vi "Test 3 Compatible Game.vi"(8 "error in (no error)":errorcluster, 11 "Test Case In":refnum<class "Game Test.lvclass">) -> (0 "error out":errorcluster, 3 "Test Case Out":refnum<class "Game Test.lvclass">)   [LabVIEW 2020, in "Game Test.lvclass"]
uses:
  Game Test.lvclass
  C:/Program Files (x86)/National Instruments/LabVIEW 2020/vi.lib/Astemes/LUnit/Test Case.lvclass
  Bag/Cubes.ctl
  <vilib>/Astemes/LUnit/Test Case.lvclass/Test Case.ctl
  <vilib>/Astemes/LUnit/Append Fail Result.vi
  <vilib>/Astemes/LUnit/Append Pass Result.vi
  Bag/Bag.lvclass
  <vilib>/Astemes/LUnit/Test Case.lvclass
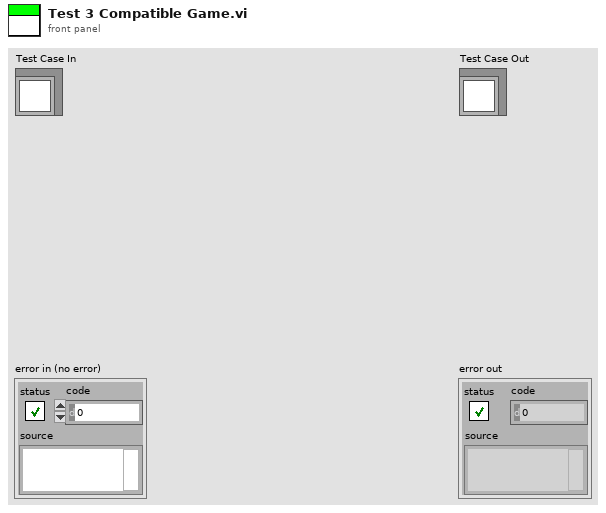
[diagram p1: front panel]
types:
  T1 = typedef "Bag.lvclass/Cubes.ctl" = cluster{"Red":i32, "Green":i32, "Blue":i32}
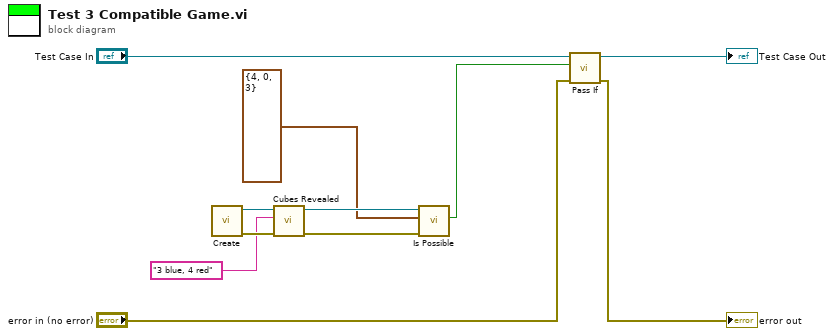
[diagram p0: block diagram]
diagram:
  n1 = call "Create.vi"() -> ("error out"=w6:errorcluster, "Bag"=w7:refnum<class "Bag.lvclass">)  [unwired: 10 in]
  n2 = call "Cubes Revealed.vi"("error in (no error)"=w6, "Set"="3 blue, 4 red", "Bag in"=w7) -> ("error out"=w3:errorcluster, "Bag out"=w4:refnum<class "Bag.lvclass">)  [unwired: 7 in]
  n3 = call "Is Possible.vi"("error in (no error)"=w3, "Cubes"=T1 {"Red"=4, "Green"=0, "Blue"=3}, "Bag in"=w4) -> ("Compatible?"=w1:bool)  [unwired: 6 in, 2 out]
  n4 = call <vilib>:"Pass If.vi"("error in (no error)"="error in (no error)", "Pass?"=w1, "LUnit Test Case In"="Test Case In") -> ("error out"=→"error out":errorcluster, "LUnit Test Case Out"=→"Test Case Out":refnum<class "Game Test.lvclass">)  [unwired: 7 in]
